vi "CustomUDPComm.vi"(8 "error in (no error)":errorcluster, 11 "connection ID":refnum<k16>) -> (3 "Autonomous":string)   [LabVIEW 2015]
uses:
  AutoVars.vi
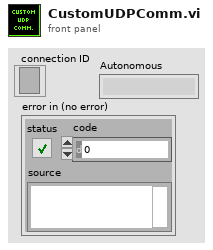
[diagram p1: front panel]
types:
  T1 = enum16{"Low Bar", "Ramparts", "Moat", "Rock Wall", "Rough Terrain", "Portcullis", "Cheval de Frise", "Drawbridge", "Sally Port"}
  T2 = enum16{"Far Left", "Pos 2", "Pos 3", "Pos 4", "Far Right"}
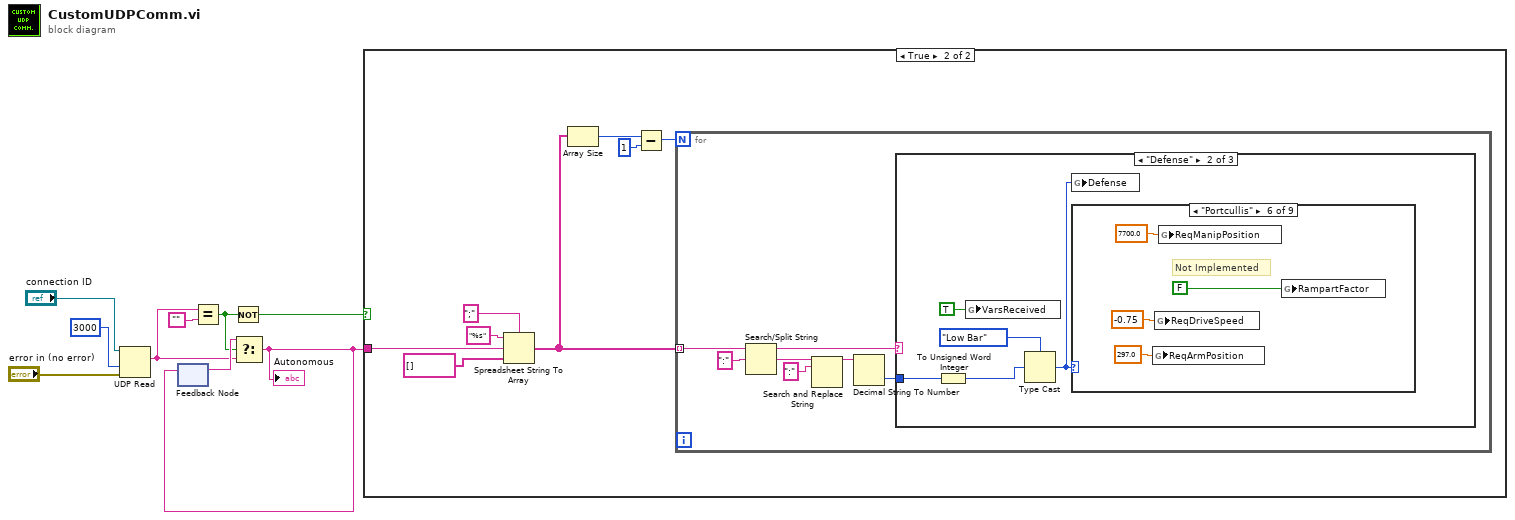
[diagram p0: block diagram]
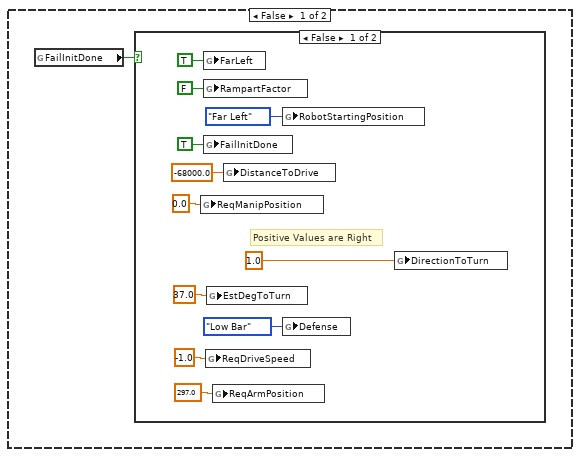
[diagram p2: hidden frame]
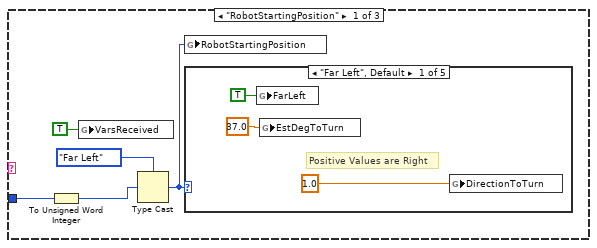
[diagram p4: hidden frame]
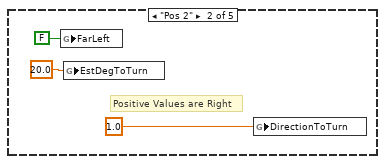
[diagram p5: hidden frame]
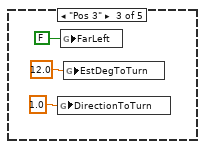
[diagram p6: hidden frame]
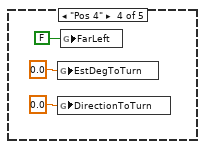
[diagram p7: hidden frame]
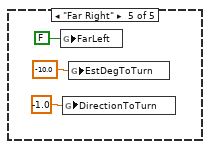
[diagram p8: hidden frame]
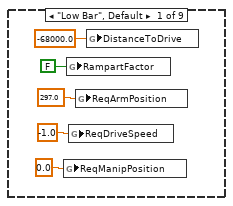
[diagram p9: hidden frame]
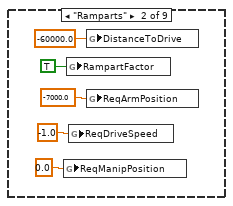
[diagram p10: hidden frame]
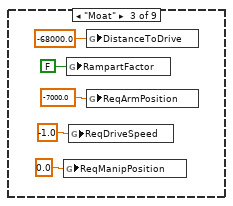
[diagram p11: hidden frame]
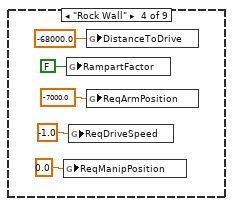
[diagram p12: hidden frame]
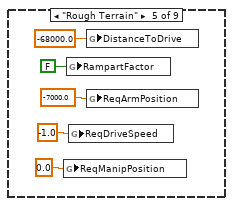
[diagram p13: hidden frame]
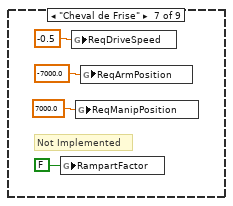
[diagram p14: hidden frame]
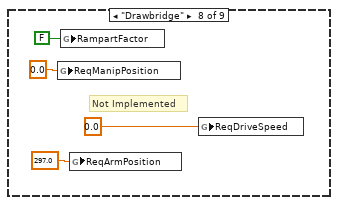
[diagram p15: hidden frame]
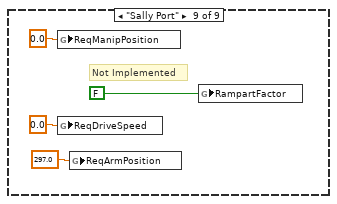
[diagram p16: hidden frame]
diagram:
  n1 = UDP Read(connection ID="connection ID", timeout ms (25000)=3000, 8:"error in (no error)") -> (data out=w5:string)  [unwired: 1 in, 4 out]
  n2 = feedback #1() -> (w6:string)  [unwired: 1 in]
  n3 = Equal?(x=w5, y="") -> (x = y?=w2:bool)
  n4 = Not(x=w2) -> (.not. x?=w1:bool)
  n5 = Select(t=w6, s=w2, f=w5) -> (s? t:f=w3:string)
  "Autonomous" <- w3
  n6 = feedback-in #1(w3) -> ()
  n7 = case shown="True" w1 {
    tunnel: w3 -> [_ w29]
    frame False {
      n8 = global read "AutoVars.vi" "FailInitDone"() -> (w10:bool)
      n9 = case shown="False" w10 {
        frame False {
          # "Positive Values are Right"
          n10 = global write "AutoVars.vi" "ReqManipPosition"(0.0 ("ReqManipPosition")) -> ()
          n11 = global write "AutoVars.vi" "FarLeft"(TRUE ("VarsReceived")) -> ()
          n12 = global write "AutoVars.vi" "RampartFactor"(FALSE ("RampartFactor")) -> ()
          n13 = global write "AutoVars.vi" "FailInitDone"(TRUE ("InitDone")) -> ()
          n14 = global write "AutoVars.vi" "ReqDriveSpeed"(-1.0 ("ReqDriveSpeed")) -> ()
          n15 = global write "AutoVars.vi" "EstDegToTurn"(37.0 ("DegToTurn")) -> ()
          n16 = global write "AutoVars.vi" "ReqArmPosition"(297.0 ("DistanceToDrive")) -> ()
          n17 = global write "AutoVars.vi" "DistanceToDrive"(-68000.0 ("DistanceToDrive")) -> ()
          n18 = global write "AutoVars.vi" "RobotStartingPosition"(T2."Far Left" ("RobotStartingPosition")) -> ()
          n19 = global write "AutoVars.vi" "Defense"(T1."Low Bar" ("Defense")) -> ()
          n20 = global write "AutoVars.vi" "DirectionToTurn"(1.0 ("DegToTurn")) -> ()
        }
        frame True {
        }
      }
    }
    frame True {
      n21 = Spreadsheet String To Array(delimiter (Tab)=";" ("search string/char (-)"), format string="%s", spreadsheet string=w29, array type (2D Dbl)=string[] []) -> (array=w25:string[])
      n22 = Array Size(array=w25) -> (size(s)=w24:i32)
      n23 = Subtract(x=w24, y=1) -> (x-y=w22:i32)
      n24 = for {
        N: w22 -> [_]
        tunnel: w25 -> [w36] mode=indexing
        n25 = Search/Split String(string=w36, search string/char (-)=":") -> (substring before match=w34:string, match + rest of string=w33:string)  [unwired: 1 in, 1 out]
        n26 = Search and Replace String(input string=w33, search string=":" ("replace string (\"\")")) -> (result string=w31:string)  [unwired: 6 in, 3 out]
        n27 = Decimal String To Number(string=w31) -> (number=w30:i32)  [unwired: 2 in, 1 out]
        n28 = case shown="\"Defense\"" w34 {
          tunnel: w30 -> [w39 w59 _]
          frame "RobotStartingPosition" {
            n29 = To Unsigned Word Integer(number=w39) -> (unsigned 16bit integer=w38:u16)
            n30 = global write "AutoVars.vi" "VarsReceived"(TRUE ("VarsReceived")) -> ()
            n31 = Type Cast(type=T2."Far Left" ("RobotStartingPosition"), x=w38) -> (*(type *) &x=w37:T2)
            n32 = global write "AutoVars.vi" "RobotStartingPosition"(w37) -> ()
            n33 = case shown="\"Far Left\", Default" w37 {
              frame "Far Left", Default {
                # "Positive Values are Right"
                n34 = global write "AutoVars.vi" "FarLeft"(TRUE ("VarsReceived")) -> ()
                n35 = global write "AutoVars.vi" "EstDegToTurn"(37.0 ("DegToTurn")) -> ()
                n36 = global write "AutoVars.vi" "DirectionToTurn"(1.0 ("DegToTurn")) -> ()
              }
              frame "Pos 2" {
                # "Positive Values are Right"
                n37 = global write "AutoVars.vi" "FarLeft"(FALSE ("VarsReceived")) -> ()
                n38 = global write "AutoVars.vi" "EstDegToTurn"(20.0 ("DegToTurn")) -> ()
                n39 = global write "AutoVars.vi" "DirectionToTurn"(1.0 ("DegToTurn")) -> ()
              }
              frame "Pos 3" {
                n40 = global write "AutoVars.vi" "DirectionToTurn"(1.0 ("DegToTurn")) -> ()
                n41 = global write "AutoVars.vi" "FarLeft"(FALSE ("VarsReceived")) -> ()
                n42 = global write "AutoVars.vi" "EstDegToTurn"(12.0 ("DegToTurn")) -> ()
              }
              frame "Pos 4" {
                n43 = global write "AutoVars.vi" "EstDegToTurn"(0.0 ("DegToTurn")) -> ()
                n44 = global write "AutoVars.vi" "DirectionToTurn"(0.0 ("DegToTurn")) -> ()
                n45 = global write "AutoVars.vi" "FarLeft"(FALSE ("VarsReceived")) -> ()
              }
              frame "Far Right" {
                n46 = global write "AutoVars.vi" "FarLeft"(FALSE ("VarsReceived")) -> ()
                n47 = global write "AutoVars.vi" "DirectionToTurn"(-1.0 ("DegToTurn")) -> ()
                n48 = global write "AutoVars.vi" "EstDegToTurn"(-10.0 ("DegToTurn")) -> ()
              }
            }
          }
          frame "Defense" {
            n49 = To Unsigned Word Integer(number=w59) -> (unsigned 16bit integer=w58:u16)
            n50 = global write "AutoVars.vi" "VarsReceived"(TRUE ("VarsReceived")) -> ()
            n51 = Type Cast(type=T1."Low Bar" ("Defense"), x=w58) -> (*(type *) &x=w57:T1)
            n52 = global write "AutoVars.vi" "Defense"(w57) -> ()
            n53 = case shown="\"Portcullis\"" w57 {
              frame "Low Bar", Default {
                n54 = global write "AutoVars.vi" "ReqManipPosition"(0.0 ("ReqManipPosition")) -> ()
                n55 = global write "AutoVars.vi" "RampartFactor"(FALSE ("RampartFactor")) -> ()
                n56 = global write "AutoVars.vi" "ReqDriveSpeed"(-1.0 ("DistanceToDrive")) -> ()
                n57 = global write "AutoVars.vi" "ReqArmPosition"(297.0 ("DistanceToDrive")) -> ()
                n58 = global write "AutoVars.vi" "DistanceToDrive"(-68000.0 ("DistanceToDrive")) -> ()
              }
              frame "Ramparts" {
                n59 = global write "AutoVars.vi" "ReqManipPosition"(0.0 ("ReqManipPosition")) -> ()
                n60 = global write "AutoVars.vi" "RampartFactor"(TRUE ("VarsReceived")) -> ()
                n61 = global write "AutoVars.vi" "ReqDriveSpeed"(-1.0 ("DistanceToDrive")) -> ()
                n62 = global write "AutoVars.vi" "DistanceToDrive"(-60000.0 ("DistanceToDrive")) -> ()
                n63 = global write "AutoVars.vi" "ReqArmPosition"(-7000.0 ("DistanceToDrive")) -> ()
              }
              frame "Moat" {
                n64 = global write "AutoVars.vi" "ReqManipPosition"(0.0 ("ReqManipPosition")) -> ()
                n65 = global write "AutoVars.vi" "RampartFactor"(FALSE ("VarsReceived")) -> ()
                n66 = global write "AutoVars.vi" "ReqDriveSpeed"(-1.0 ("DistanceToDrive")) -> ()
                n67 = global write "AutoVars.vi" "DistanceToDrive"(-68000.0 ("DistanceToDrive")) -> ()
                n68 = global write "AutoVars.vi" "ReqArmPosition"(-7000.0 ("DistanceToDrive")) -> ()
              }
              frame "Rock Wall" {
                n69 = global write "AutoVars.vi" "ReqManipPosition"(0.0 ("ReqManipPosition")) -> ()
                n70 = global write "AutoVars.vi" "RampartFactor"(FALSE ("RampartFactor")) -> ()
                n71 = global write "AutoVars.vi" "ReqDriveSpeed"(-1.0 ("DistanceToDrive")) -> ()
                n72 = global write "AutoVars.vi" "DistanceToDrive"(-68000.0 ("DistanceToDrive")) -> ()
                n73 = global write "AutoVars.vi" "ReqArmPosition"(-7000.0 ("DistanceToDrive")) -> ()
              }
              frame "Rough Terrain" {
                n74 = global write "AutoVars.vi" "ReqManipPosition"(0.0 ("ReqManipPosition")) -> ()
                n75 = global write "AutoVars.vi" "RampartFactor"(FALSE ("RampartFactor")) -> ()
                n76 = global write "AutoVars.vi" "ReqDriveSpeed"(-1.0 ("DistanceToDrive")) -> ()
                n77 = global write "AutoVars.vi" "DistanceToDrive"(-68000.0 ("DistanceToDrive")) -> ()
                n78 = global write "AutoVars.vi" "ReqArmPosition"(-7000.0 ("DistanceToDrive")) -> ()
              }
              frame "Portcullis" {
                # "Not Implemented"
                n79 = global write "AutoVars.vi" "ReqArmPosition"(297.0 ("DistanceToDrive")) -> ()
                n80 = global write "AutoVars.vi" "ReqDriveSpeed"(-0.75 ("DistanceToDrive")) -> ()
                n81 = global write "AutoVars.vi" "ReqManipPosition"(7700.0 ("ReqManipPosition")) -> ()
                n82 = global write "AutoVars.vi" "RampartFactor"(FALSE ("RampartFactor")) -> ()
              }
              frame "Cheval de Frise" {
                # "Not Implemented"
                n83 = global write "AutoVars.vi" "RampartFactor"(FALSE ("RampartFactor")) -> ()
                n84 = global write "AutoVars.vi" "ReqDriveSpeed"(-0.5 ("DistanceToDrive")) -> ()
                n85 = global write "AutoVars.vi" "ReqManipPosition"(7000.0 ("ReqManipPosition")) -> ()
                n86 = global write "AutoVars.vi" "ReqArmPosition"(-7000.0 ("DistanceToDrive")) -> ()
              }
              frame "Drawbridge" {
                # "Not Implemented"
                n87 = global write "AutoVars.vi" "ReqManipPosition"(0.0 ("ReqManipPosition")) -> ()
                n88 = global write "AutoVars.vi" "RampartFactor"(FALSE ("RampartFactor")) -> ()
                n89 = global write "AutoVars.vi" "ReqArmPosition"(297.0 ("DistanceToDrive")) -> ()
                n90 = global write "AutoVars.vi" "ReqDriveSpeed"(0.0 ("DistanceToDrive")) -> ()
              }
              frame "Sally Port" {
                # "Not Implemented"
                n91 = global write "AutoVars.vi" "ReqManipPosition"(0.0 ("ReqManipPosition")) -> ()
                n92 = global write "AutoVars.vi" "ReqDriveSpeed"(0.0 ("DistanceToDrive")) -> ()
                n93 = global write "AutoVars.vi" "ReqArmPosition"(297.0 ("DistanceToDrive")) -> ()
                n94 = global write "AutoVars.vi" "RampartFactor"(FALSE ("RampartFactor")) -> ()
              }
            }
          }
          frame "False", Default {
          }
        }
      }
    }
  }
